vi "Analysis.Result Summaries, First and Last Pass Yield Paretos_V3.vi"(11 "ResultSum":T2[](array[typedef])) -> (0 "Dur Hist":T1(graph), 1 "Durs":string[][](table), 2 "Test Count Table":string[][](table), 3 "Failure Pareto":string[][](table))   [LabVIEW 2024]
uses:
  Analysis.Result Summary.ctl
panel:
  out "Tst Cnts":i32
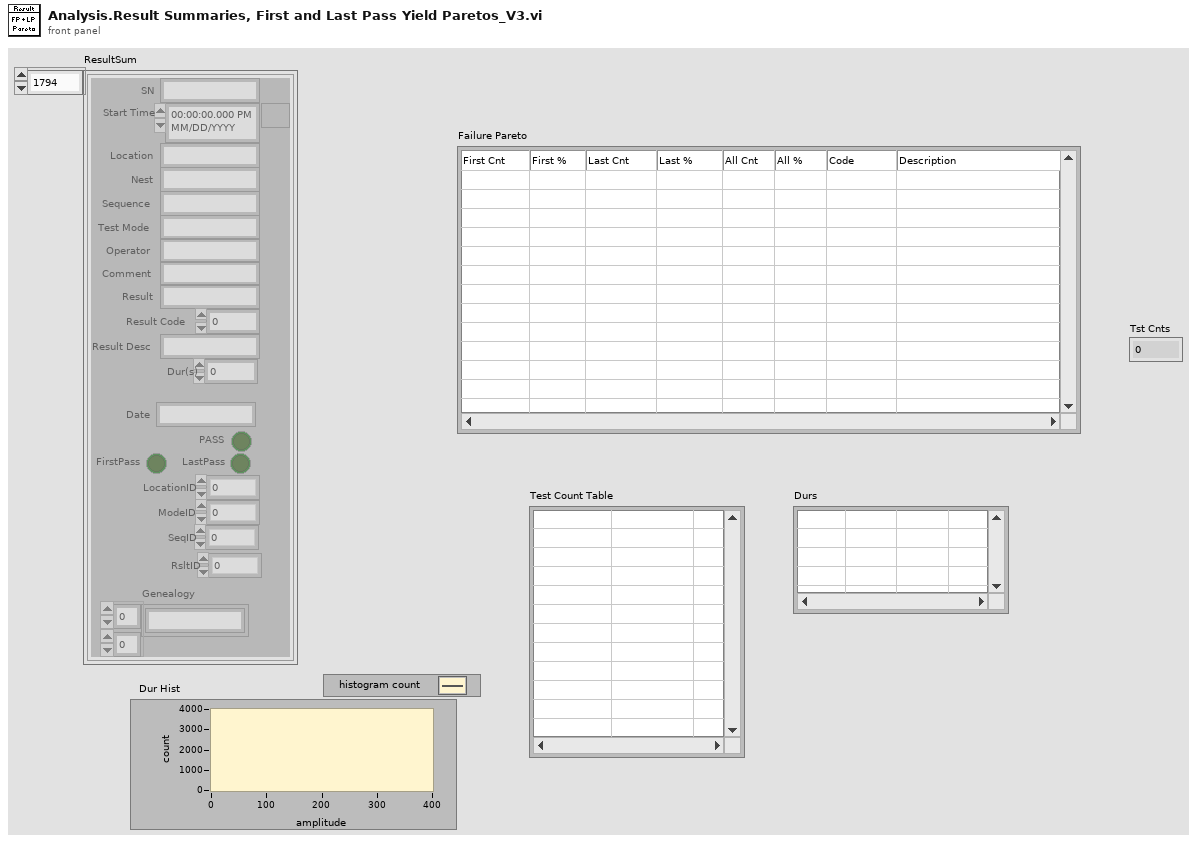
[diagram p1: front panel]
types:
  T1 = cluster{"X Values":dbl[], "Histogram: h(x)":i32[]}
  T2 = typedef "Analysis.Result Summary.ctl" = cluster{"SN":string, "Start Time":timestamp, "Location":string, "Nest":string, "Sequence":string, "Operator":string, "Test Mode":string, "Comment":string, "Result":string, "Result Code":i32, "Result Desc":string, "Date":string, "Dur(s)":dbl, "PASS":bool, "FirstPass":bool, "LastPass":bool, "LocationID":i32, "ModeID":i32, "SeqID":i32, "RsltID":i32, "Genealogy":string[][]}
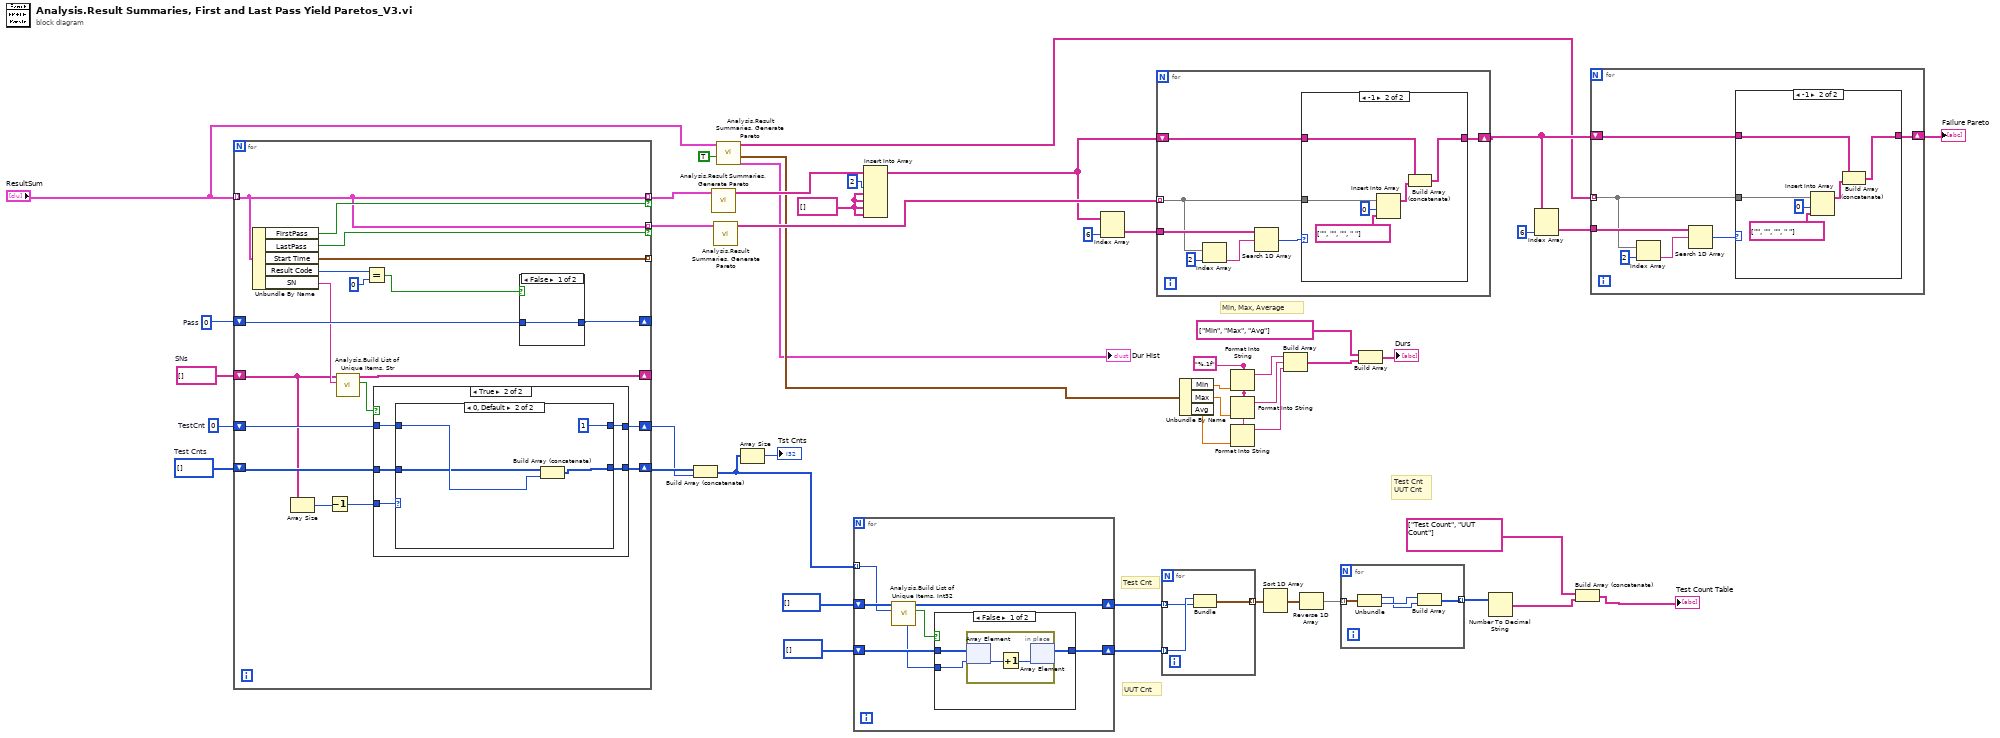
[diagram p0: block diagram]
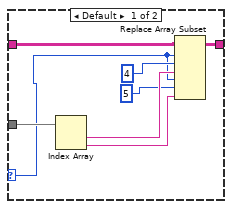
[diagram p2: hidden frame]
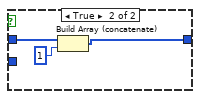
[diagram p3: hidden frame]
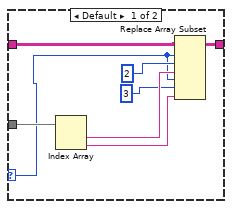
[diagram p4: hidden frame]
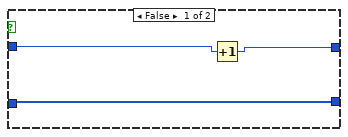
[diagram p5: hidden frame]
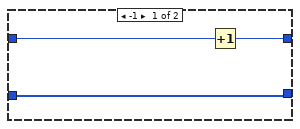
[diagram p6: hidden frame]
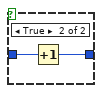
[diagram p7: hidden frame]
diagram:
  w17 = "%.1f"
  w9 = string[] []
  w43 = string[] []  # SNs
  w45 = i32[] []  # Test Cnts
  w44 = 0  # TestCnt
  w46 = 0  # Pass
  # "Min, Max, Average"
  # "Test Cnt\nUUT Cnt"
  # "Test Cnt"
  # "UUT Cnt"
  n1 = for {
    tunnel: "ResultSum" -> [w63] mode=indexing
    tunnel: [w63] -> w32 mode=indexing if=w66
    tunnel: [w63] -> w47 mode=indexing if=w65
    tunnel: [w64] -> _ mode=indexing
    shift-right: [w60] -> _
    shift-left: w46 -> [w58]
    shift-right: [w52] -> w42
    shift-left: w45 -> [w54]
    shift-right: [w53] -> w41
    shift-left: w44 -> [w51]
    shift-right: [w56] -> _
    shift-left: w43 -> [w50]
    n2 = Unbundle By Name(w63) -> ("FirstPass"=w66:bool, "LastPass"=w65:bool, "Start Time"=w64:timestamp, "Result Code"=w62:i32, "SN"=w57:string)
    n3 = Array Size(array=w50) -> (size(s)=w49:i32)
    n4 = Decrement(x=w49) -> (x-1=w48:i32)
    n5 = call "Analysis.Build List of Unique Items, Str.vi"("Item In"=w57, "List In"=w50) -> ("Added"=w55:bool, "List Out"=w56:string[])  [unwired: 7 in, 1 out]
    n6 = Equal?(x=w62, y=0) -> (x = y?=w59:bool)
    n7 = case shown="True" w55 {
      tunnel: w54 -> [w69 w71]
      tunnel: w51 -> [w68 w72]
      tunnel: [w67 w74] -> w53
      tunnel: [w69 w73] -> w52
      tunnel: w48 -> [_ w70]
      frame False {
        n8 = Increment(x=w68) -> (x+1=w67:i32)
      }
      frame True {
        n9 = case shown="0, Default" w70 {
          tunnel: [w75 1] -> w74
          tunnel: [w77 w80] -> w73
          tunnel: w72 -> [w76 w79]
          tunnel: w71 -> [w77 w78]
          frame -1 {
            n10 = Increment(x=w76) -> (x+1=w75:i32)
          }
          frame 0, Default {
            n11 = Build Array (concatenate)(w78, w79) -> (w80:i32[])
          }
        }
      }
    }
    n12 = case shown="False" w59 {
      tunnel: w58 -> [w82 w84]
      tunnel: [w82 w83] -> w60
      frame False {
      }
      frame True {
        n13 = Increment(x=w84) -> (x+1=w83:i32)
      }
    }
  }
  n14 = Build Array (concatenate)(w42, w41) -> (w33:i32[])
  n15 = call "Analysis.Result Summaries, Generate Pareto.vi"("ResultSum"=w32) -> ("FP Pareto"=w38:string[][])  [unwired: 7 in, 3 out]
  n16 = call "Analysis.Result Summaries, Generate Pareto.vi"("ResultSum"=w47) -> ("FP Pareto"=w39:string[][])  [unwired: 7 in, 3 out]
  n17 = call "Analysis.Result Summaries, Generate Pareto.vi"("Calc Duration"=TRUE, "ResultSum"="ResultSum") -> ("Test Time Histogram"=→"Dur Hist":T1, "Test Times (s)"=w3:cluster{"Min":dbl, "Max":dbl, "Avg":dbl}, "FP Pareto"=w4:string[][])  [unwired: 6 in, 1 out]
  n18 = Array Size(array=w33) -> (size(s)=→"Tst Cnts":i32)
  n19 = for {
    tunnel: w33 -> [w89] mode=indexing
    shift-right: [w90] -> w29
    shift-left: i32[] [] ("Test Cnts") -> [w91]
    shift-right: [w86] -> w28
    shift-left: i32[] [] ("Test Cnts") -> [w87]
    n20 = call "Analysis.Build List of Unique Items, Int32.vi"("Item In"=w89, "List In"=w91) -> ("Added"=w88:bool, "List Out"=w90:i32[], "Index"=w85:i32)  [unwired: 7 in]
    n21 = case shown="False" w88 {
      tunnel: w87 -> [w94 w98]
      tunnel: [w93 w99] -> w86
      tunnel: w85 -> [w92 _]
      frame False {
        n22 = in-place {
          n23 = in-place-array #1(w94, w92) -> (w96:i32)
          n24 = Increment(x=w96) -> (x+1=w95:i32)
          n25 = in-place-array #1(w95) -> (w93:i32[])  [unwired: 1 out]
        }
      }
      frame True {
        n26 = Build Array (concatenate)(w98, 1) -> (w99:i32[])
      }
    }
  }
  n27 = Insert Into Array(array=w38, index (col)=2 ("index (row)"), new element #1=w9, new element #2=w9, new element #3=w9, new element #4=w9) -> (w37:string[][])  [unwired: 1 in]
  n28 = Index Array(array=w37, index (col)=6 ("index (row)")) -> (element=w35:string[])  [unwired: 1 in]
  n29 = for {
    tunnel: w39 -> [w101] mode=indexing
    tunnel: w35 -> [w105]
    shift-right: [w100] -> w5
    shift-left: w37 -> [w103]
    n30 = Index Array(array=w101, index=2) -> (element=w104:string)
    n31 = Search 1D Array(1D array=w105, element=w104) -> (index of element=w102:i32)  [unwired: 1 in]
    n32 = case shown="-1" w102 {
      selector: w102 -> [w109 _]
      tunnel: w103 -> [w112 w120]
      tunnel: w101 -> [w114 w119]
      tunnel: [w113 w115] -> w100
      frame Default {
        n33 = Index Array(array=w114) -> (element #1=w110:string, element #2=w107:string)  [unwired: 2 in]
        n34 = Replace Array Subset(array=w112, new element #1=w110, index (row) #1=w109, index (col) #1=2 ("disabled index (col)"), new element #2=w107, index (row) #2=w109, index (col) #2=3 ("disabled index (col)")) -> (w113:string[][])
      }
      frame -1 {
        n35 = Insert Into Array(array=w119, index=0, new element=string[] ["", "", "", " "]) -> (w116:string[])
        n36 = Build Array (concatenate)(w120, w116) -> (w115:string[][])
      }
    }
  }
  n37 = for {
    tunnel: w29 -> [w122] mode=indexing
    tunnel: w28 -> [w123] mode=indexing
    tunnel: [w121] -> w27 mode=indexing
    n38 = Bundle("TestCnt"=w123, "TestCnt"=w122) -> (w121:cluster{"TestCnt":i32, "TestCnt":i32})  [unwired: 1 in]
  }
  n39 = Unbundle By Name(w3) -> ("Min"=w20:dbl, "Max"=w19:dbl, "Avg"=w18:dbl)
  n40 = Format Into String(format string=w17, w20) -> (resulting string=w16:string)  [unwired: 2 in, 1 out]
  n41 = Format Into String(format string=w17, w19) -> (resulting string=w15:string)  [unwired: 2 in, 1 out]
  n42 = Format Into String(format string=w17, w18) -> (resulting string=w14:string)  [unwired: 2 in, 1 out]
  n43 = Sort 1D Array(array=w27) -> (sorted array=w26:cluster{"TestCnt":i32, "TestCnt":i32}[])
  n44 = Build Array(w16, w15, w14) -> (w12:string[])
  n45 = Reverse 1D Array(array=w26) -> (reversed array=w25:cluster{"TestCnt":i32, "TestCnt":i32}[])
  n46 = for {
    tunnel: w25 -> [w127] mode=indexing
    tunnel: [w124] -> w24 mode=indexing
    n47 = Unbundle(w127) -> ("TestCnt"=w125:i32, "TestCnt"=w126:i32)
    n48 = Build Array(w126, w125) -> (w124:i32[])
  }
  n49 = Build Array(string[] ["Min", "Max", "Avg"], w12) -> (→"Durs":string[][])
  n50 = Number To Decimal String(number=w24) -> (decimal integer string=w21:string[][])  [unwired: 1 in]
  n51 = Index Array(array=w5, index (col)=6 ("index (row)")) -> (element=w8:string[])  [unwired: 1 in]
  n52 = Build Array (concatenate)(string[] ["Test Count", "UUT Count"], w21) -> (→"Test Count Table":string[][])
  n53 = for {
    tunnel: w4 -> [w129] mode=indexing
    tunnel: w8 -> [w133]
    shift-right: [w128] -> w6
    shift-left: w5 -> [w131]
    n54 = Index Array(array=w129, index=2) -> (element=w132:string)
    n55 = Search 1D Array(1D array=w133, element=w132) -> (index of element=w130:i32)  [unwired: 1 in]
    n56 = case shown="-1" w130 {
      selector: w130 -> [w137 _]
      tunnel: w131 -> [w140 w148]
      tunnel: w129 -> [w142 w147]
      tunnel: [w141 w143] -> w128
      frame Default {
        n57 = Index Array(array=w142) -> (element #1=w138:string, element #2=w135:string)  [unwired: 2 in]
        n58 = Replace Array Subset(array=w140, new element #1=w138, index (row) #1=w137, index (col) #1=4 ("disabled index (col)"), new element #2=w135, index (row) #2=w137, index (col) #2=5 ("disabled index (col)")) -> (w141:string[][])
      }
      frame -1 {
        n59 = Insert Into Array(array=w147, index=0, new element=string[] ["", "", "", " "]) -> (w144:string[])
        n60 = Build Array (concatenate)(w148, w144) -> (w143:string[][])
      }
    }
  }
  "Failure Pareto" <- w6
